vi "Read Frame Range.vi"(8 "error in (no error)":errorcluster, 11 "Video File in":refnum<class "Video File.lvclass">) -> (0 "error out":errorcluster, 2 "Number of Frames":u32, 3 "Video File out":refnum<class "Video File.lvclass">)   [LabVIEW 2018, in "Video File.lvclass"]
uses:
  Video File.lvclass
  Video File.lvclass/Video File.ctl
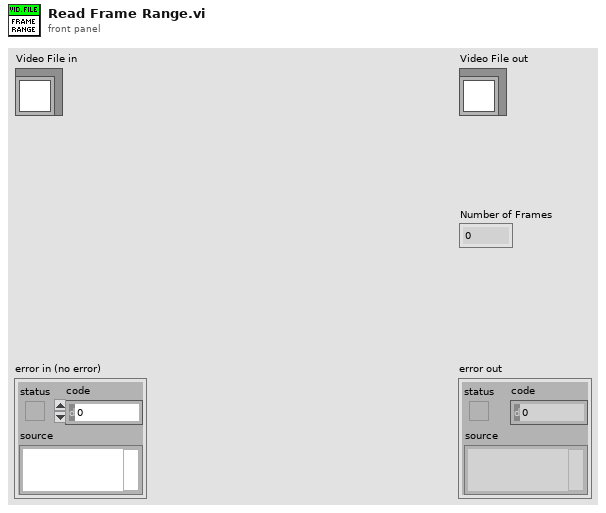
[diagram p1: front panel]
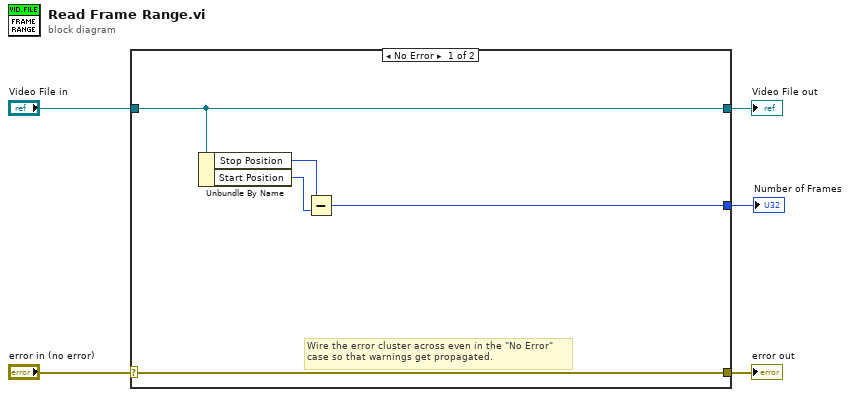
[diagram p0: block diagram]
diagram:
  n1 = case shown="No Error" "error in (no error)" {
    selector: "error in (no error)" -> [w10 w12]
    tunnel: [w10 w12] -> w4
    tunnel: [w9 w11] -> w2
    tunnel: "Video File in" -> [w9 w11]
    tunnel: [w6 _] -> w1
    frame No Error {
      # "Wire the error cluster across even in the \"No Error\"\ncase so that warnings get propagated."
      n2 = Unbundle By Name(w9) -> ("Stop Position"=w8:u32, "Start Position"=w7:u32)
      n3 = Subtract(x=w8, y=w7) -> (x-y=w6:u32)
    }
    frame Error {
    }
  }
  "error out" <- w4
  "Video File out" <- w2
  "Number of Frames" <- w1
